vi "禹山电导率校准.vi"() -> ()   [LabVIEW 2016, in "斯坦道多参数.lvlib"]
uses:
  <vilib>/Utility/miscctls.llb/LVPointTypeDef.ctl
  <vilib>/Analysis/NI_AALBase.lvlib
  <vilib>/Analysis/NI_AALPro.lvlib
  <vilib>/Utility/config.llb/NI_LVConfig.lvlib
panel:
  out "第二点校准值":dbl
  out "第一点校准值":dbl
  out "最小值":sgl format="%.2g"
  out "最大值":sgl format="%.2g"
  in  "校准停止":bool
  in  "校准模式":enum16{"两点校准", "单点校准"}(ring)
  in  "标液2":dbl
  in  "标液1":dbl
  out "波形图表":sgl(graph) caption="历史曲线"
  out "温度测量值":dbl caption="温度"
  out "变异系数":dbl format="%.6g"
  out "standard deviation":dbl caption="标准差" format="%0.2f"
  out "mean":dbl caption="均值" format="%0.2f"
  out "提示":string
  in  "校准启动":bool
  out "测试值":dbl
  out "电极斜率":dbl
  out "电极零点":dbl
  # "电导率电极设定"
  # "℃"
  # "uS/cm"
  # "请选择校准模式:"
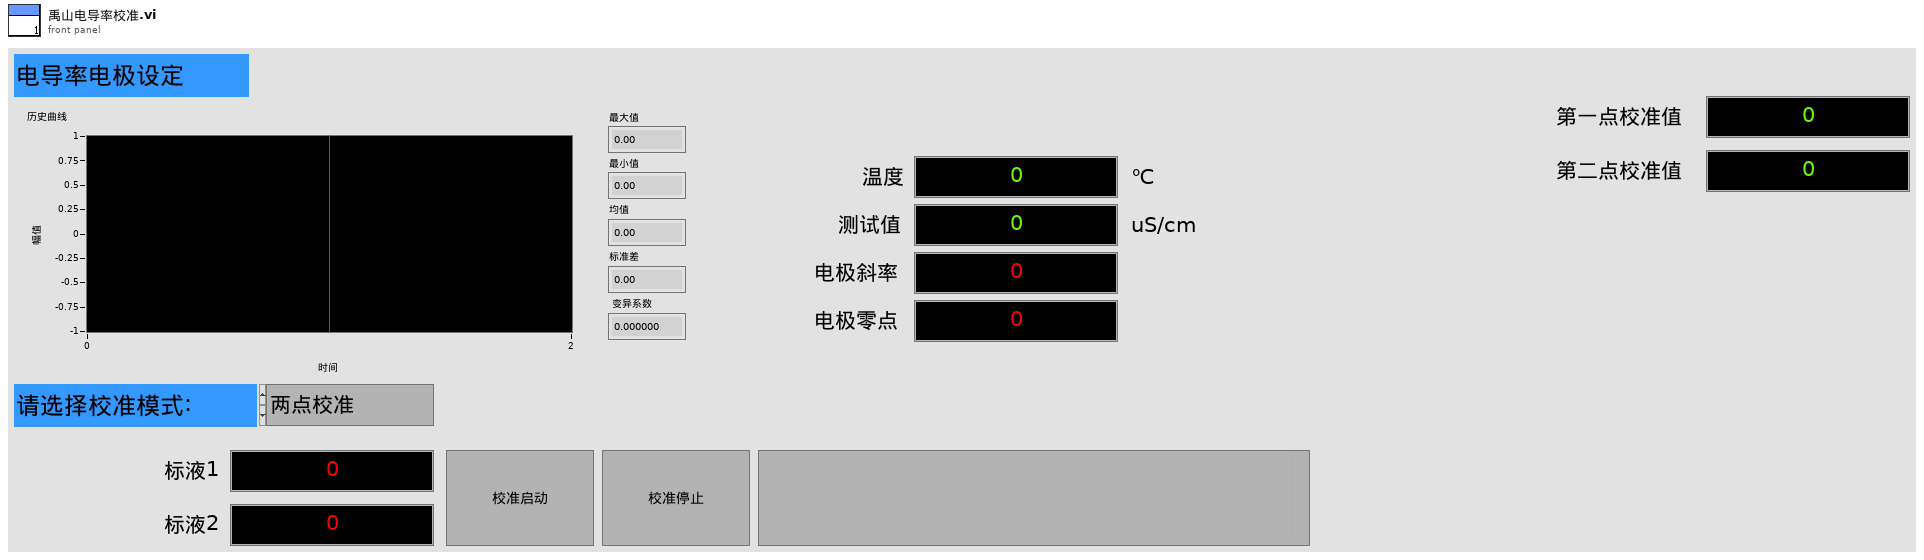
[diagram p1: front panel]
types:
  T1 = typedef "斯坦道多参数.lvlib/校准步骤.ctl" = enum16{"待机", "放置第一点标液", "第一点校准启动", "第一点校准写入", "第一点校准失败", "放置第二点标液", "第二点校准启动", "第二点校准写入", "第二点校准失败", "放置第三点标液", "第三点校准启动", "第三点校准写入", "第三点校准失败", "校准结果写入", "校准结束"}
  T2 = typedef "LVPointTypeDef.ctl" = cluster{"Horizontal":i16, "Vertical":i16}
  T3 = typedef "NI_LVConfig.lvlib/Config Data RefNum.ctl" = refnum<k1>
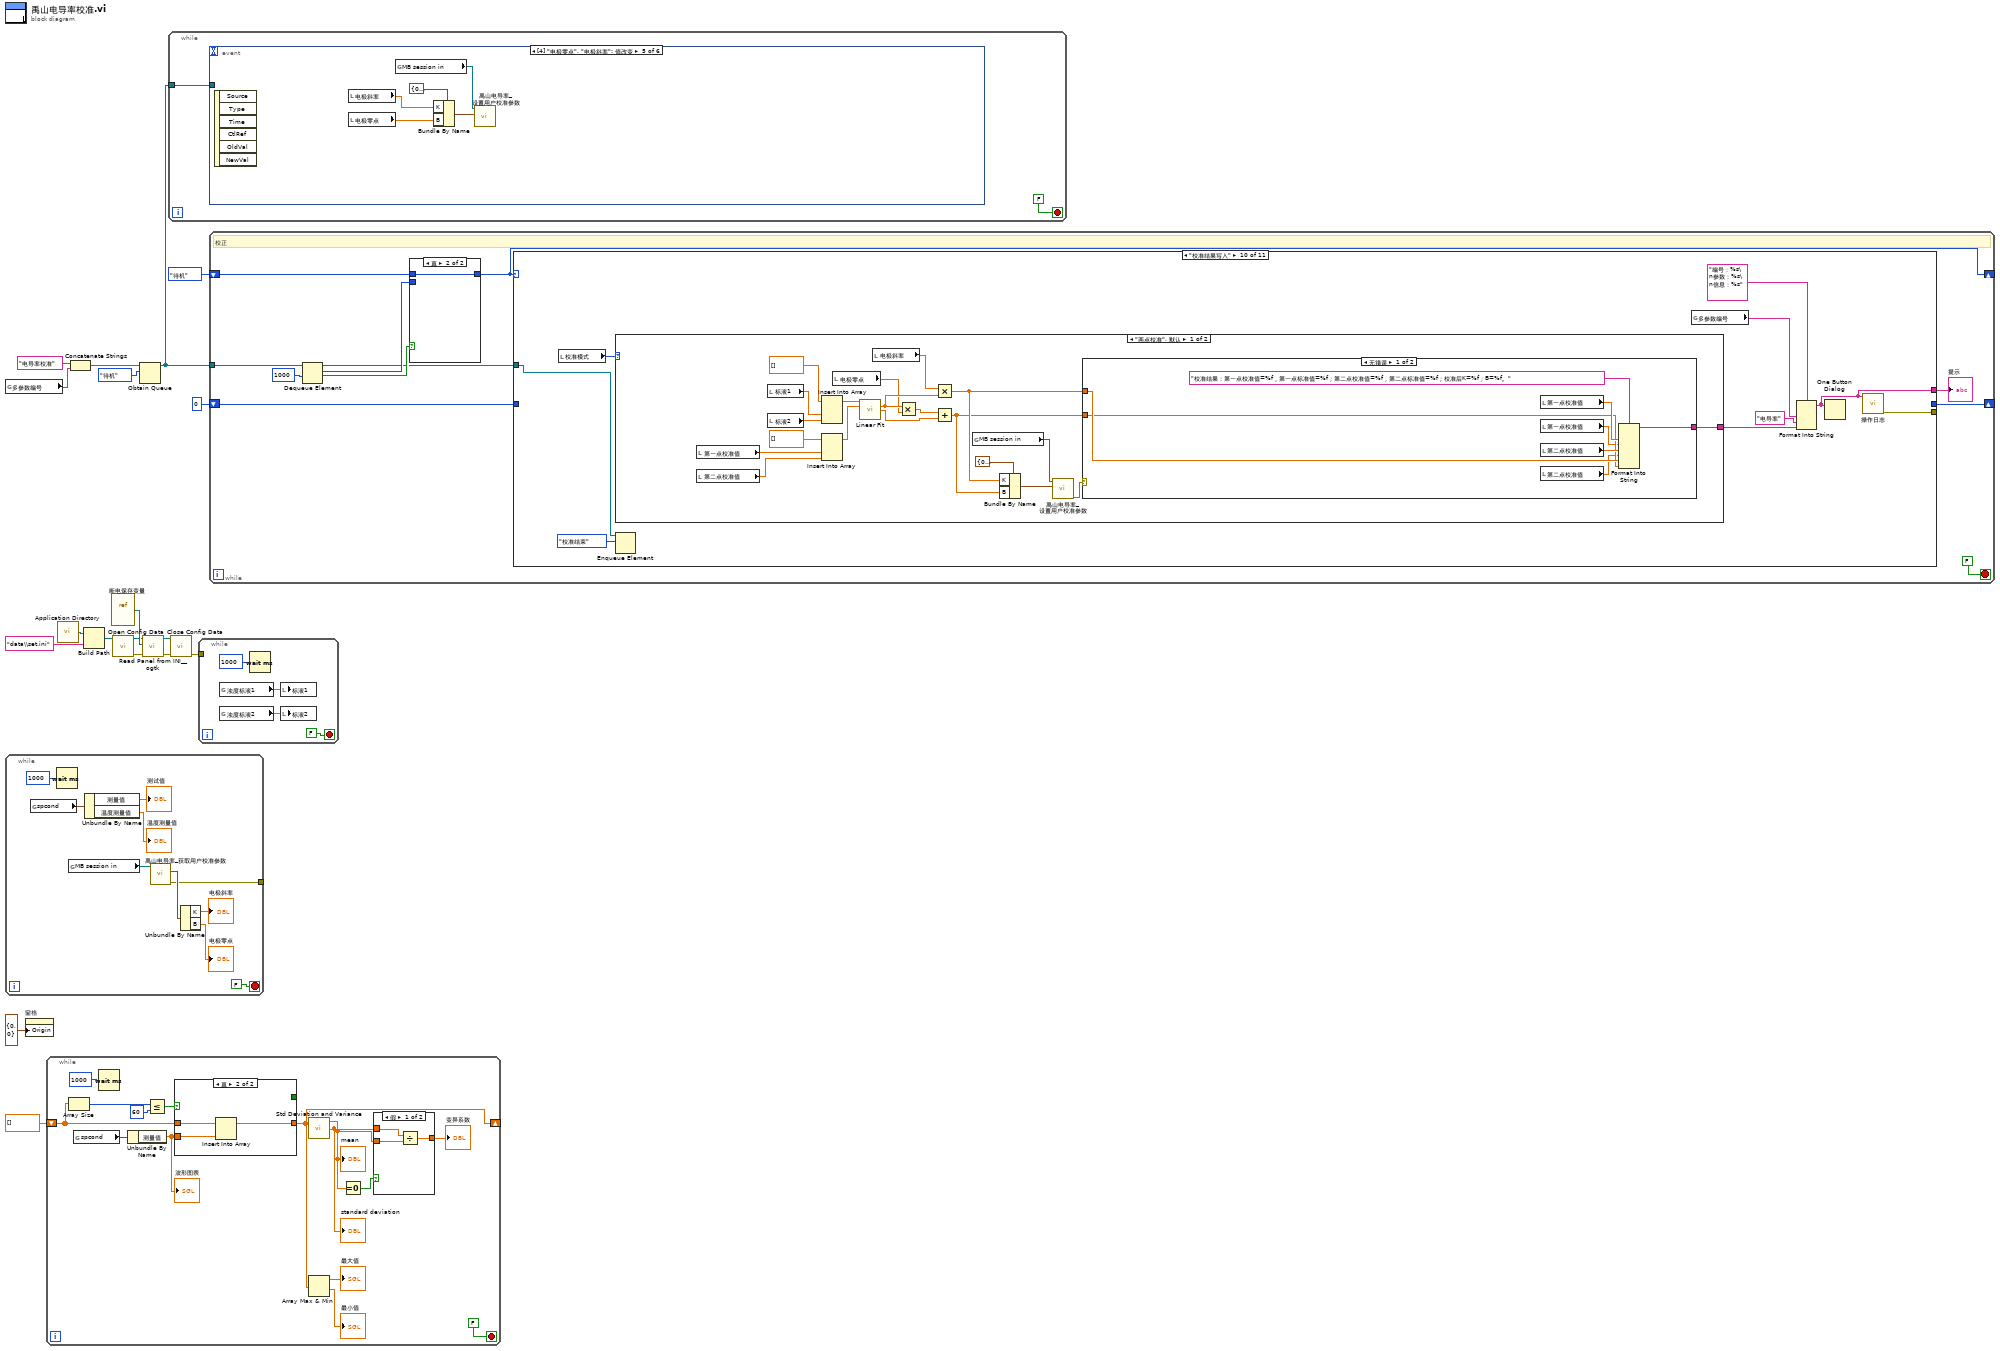
[diagram p0: block diagram]
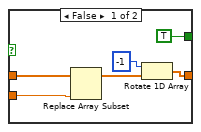
[diagram p3: hidden frame]
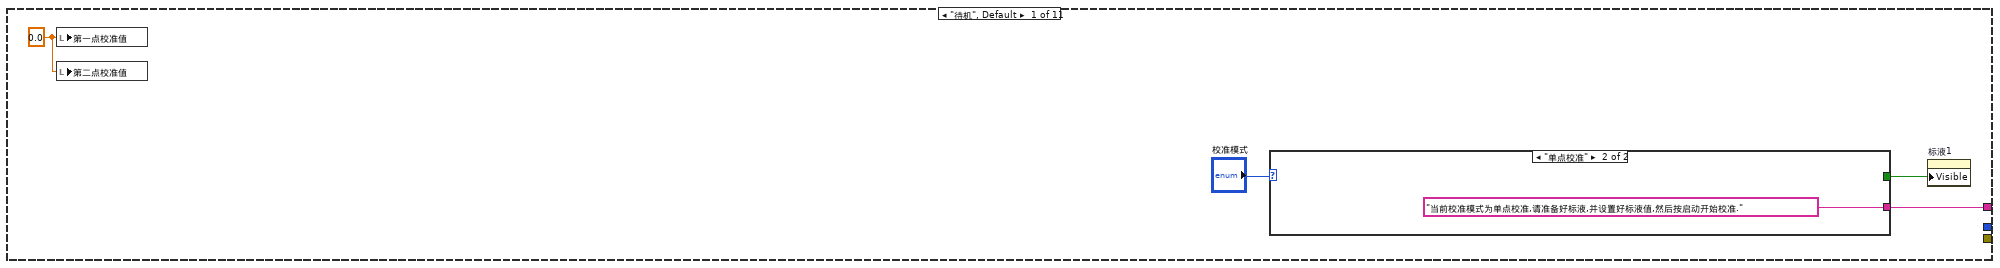
[diagram p5: hidden frame]
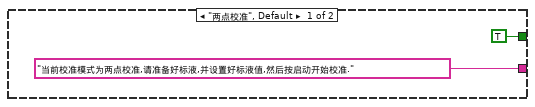
[diagram p6: hidden frame]
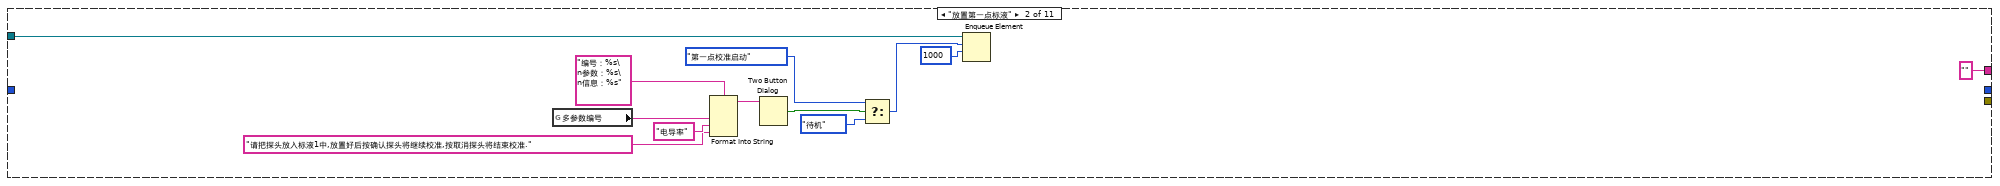
[diagram p7: hidden frame]
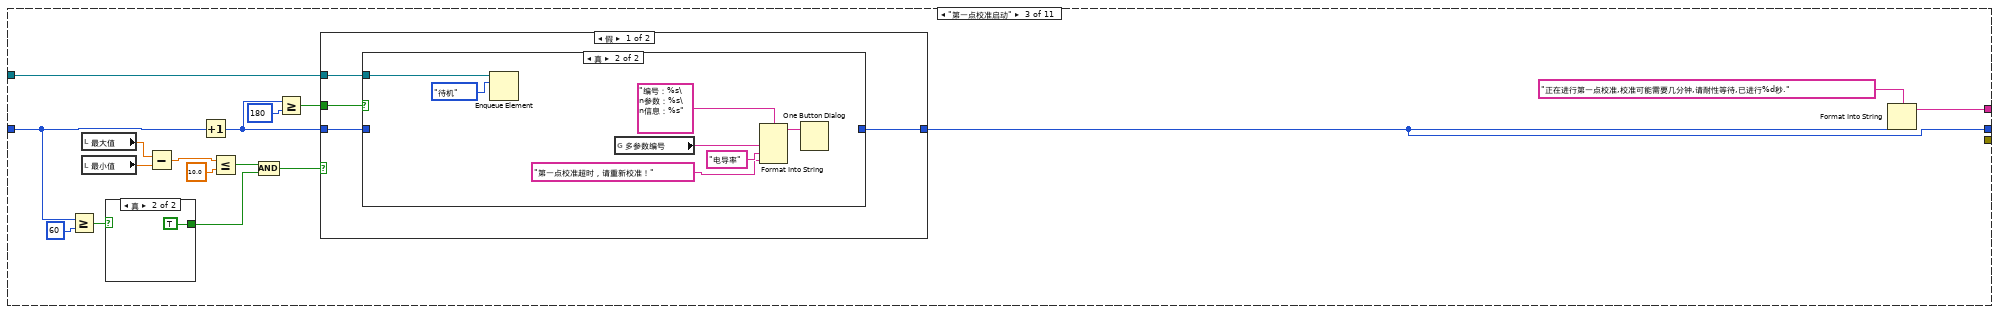
[diagram p8: hidden frame]
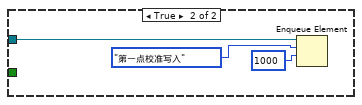
[diagram p10: hidden frame]
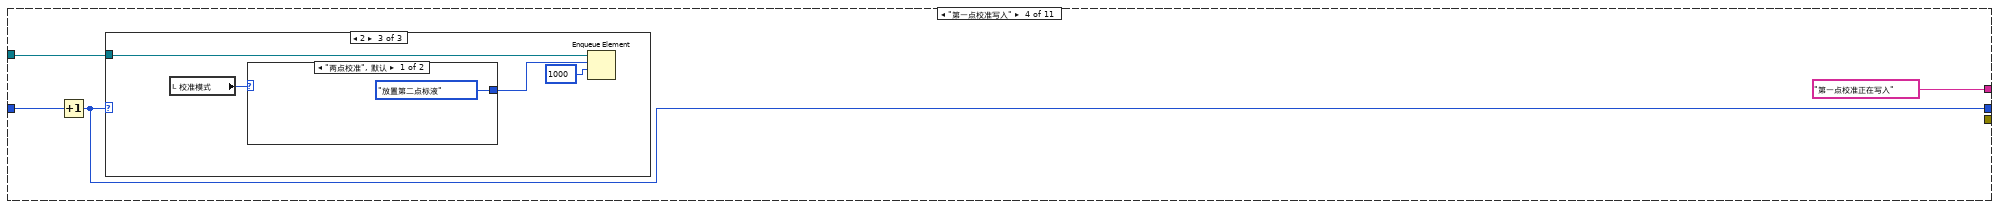
[diagram p12: hidden frame]
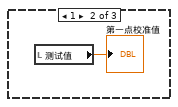
[diagram p14: hidden frame]
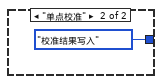
[diagram p15: hidden frame]
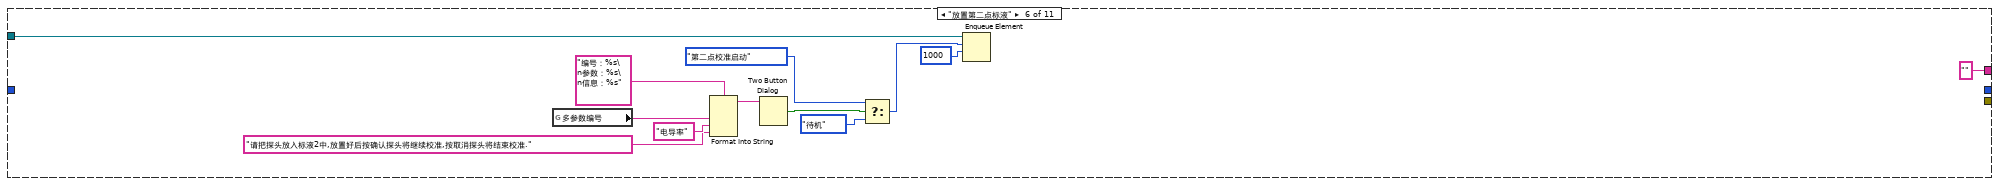
[diagram p17: hidden frame]
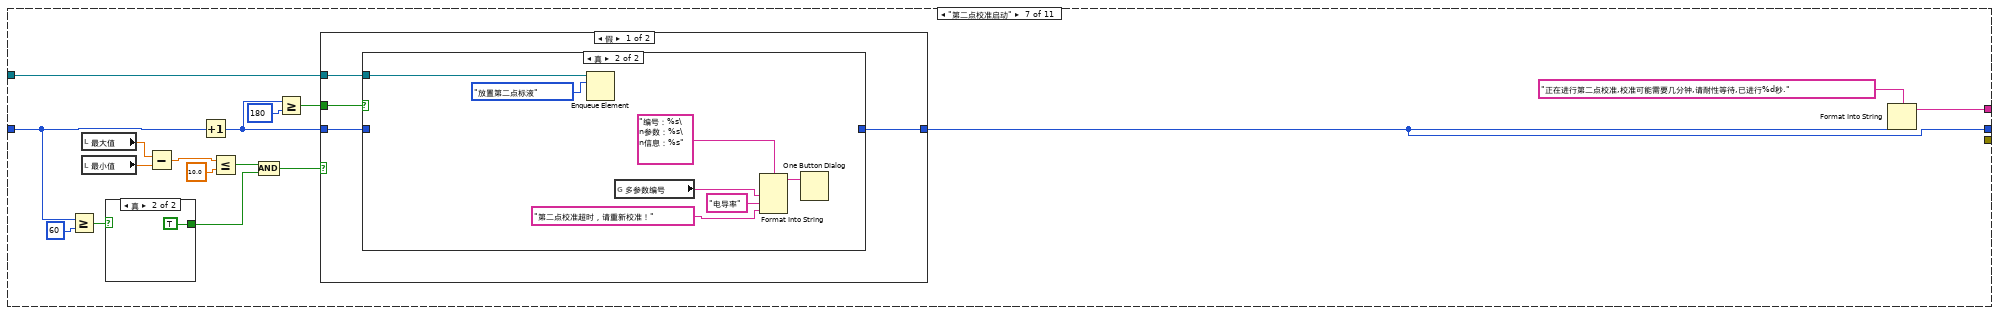
[diagram p18: hidden frame]
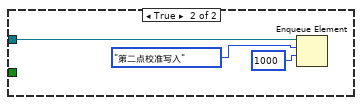
[diagram p20: hidden frame]
diagram:
  n1 = global read "多参数全局变量.vi" "多参数编号"() -> (w1:string)
  n2 = while {
    tunnel: [w23] -> _
    stop <- FALSE stop-if-true
    n3 = global read "禹山过程全局变量.vi" "spcond"() -> (w20:cluster{"温度测量值":sgl, "测量值":sgl, "错误标志":u16})
    n4 = Wait (ms)(milliseconds to wait=u32 1000 ("等待时间（毫秒）")) -> ()  [unwired: 1 out]
    n5 = global read "多参数全局变量.vi" "MB session in"() -> (w19:refnum<class "MB_Master.lvclass">)
    n6 = Unbundle By Name(w20) -> ("测量值"=→"测试值":sgl, "温度测量值"=→"温度测量值":sgl)
    n7 = call "禹山电导率_获取用户校准参数.vi"("MB session in"=w19) -> ("error out"=w23:errorcluster, "输出值"=w26:cluster{"K":sgl, "B":sgl})  [unwired: 8 in, 1 out]
    n8 = Unbundle By Name(w26) -> ("K"=→"电极斜率":sgl, "B"=→"电极零点":sgl)
  }
  n9 = property on="窗格" class="Pane"("Origin"=T2 {"Horizontal"=0, "Vertical"=0} ("原点")) -> ()  [unwired: 2 in, 2 out]
  n10 = while {
    shift-right: [w31] -> _
    shift-left: sgl[] [] -> [w39]
    stop <- FALSE stop-if-true
    n11 = Array Size(array=w39) -> (size(s)=w41:i32)
    n12 = global read "禹山过程全局变量.vi" "spcond"() -> (w33:cluster{"温度测量值":sgl, "测量值":sgl, "错误标志":u16})
    n13 = Wait (ms)(milliseconds to wait=u32 1000 ("等待时间（毫秒）")) -> ()  [unwired: 1 out]
    n14 = Unbundle By Name(w33) -> ("测量值"=w32:sgl)
    "波形图表" <- w32
    n15 = Less Or Equal?(x=w41, y=60) -> (x <= y?=w40:bool)
    n16 = case shown="真" w40 {
      tunnel: w39 -> [w52 w55]
      tunnel: w32 -> [w50 w54]
      tunnel: [w48 w53] -> w31
      tunnel: [TRUE _] -> _
      frame False {
        n17 = Replace Array Subset(array=w52, new element=w50) -> (w51:sgl[])  [unwired: 1 in]
        n18 = Rotate 1D Array(1:w51, 2:-1 ("n")) -> (0:w48:sgl[])
      }
      frame True {
        n19 = Insert Into Array(array=w55, new element=w54) -> (w53:sgl[])  [unwired: 1 in]
      }
    }
    n20 = call <vilib>:"Std Deviation and Variance.vi"("X"=w31) -> ("mean"=w34:dbl, "standard deviation"=w35:dbl)  [unwired: 1 in, 1 out]
    "standard deviation" <- w35
    "mean" <- w34
    n21 = Array Max & Min(array=w31) -> (max value=→"最大值":sgl, min value=→"最小值":sgl)  [unwired: 2 out]
    n22 = Equal To 0?(x=w34) -> (x = 0?=w38:bool)
    n23 = case shown="假" w38 {
      tunnel: w35 -> [w46 _]
      tunnel: [w45 _] -> w37
      tunnel: w34 -> [w44 _]
      frame False {
        n24 = Divide(x=w46, y=w44) -> (x/y=w45:dbl)
      }
      frame True {
      }
    }
    "变异系数" <- w37
  }
  n25 = call <vilib>:"Application Directory.vi"() -> ("Application Directory"=w8:path)
  n26 = Concatenate Strings("电导率校准" ("名称（未命名）"), w1) -> (w2:string)
  n27 = Build Path(base path=w8, name or relative path="data\\set.ini" ("名称或相对路径")) -> (appended path=w9:path)
  n28 = vi-ref "断电保存变量.vi"() -> (w11:refnum<vi>)
  n29 = call <vilib>:"Open Config Data.vi"("configuration file path"=w9) -> ("error out"=w5:errorcluster, "refnum"=w4:T3)  [unwired: 8 in, 1 out]
  n30 = Obtain Queue(name (unnamed)=w2, element data type=校准步骤."待机" ("枚举")) -> (queue out=w12:refnum<queue>)  [unwired: 3 in, 2 out]
  n31 = call <userlib>:"Read Panel from INI__ogtk.vi"("error in (no error)"=w5, "VI ref"=w11, "refnum"=w4) -> ("error out"=w7:errorcluster, "refnum out"=w6:T3)  [unwired: 7 in]
  n32 = while {
    tunnel: w12 -> [w56]
    stop <- FALSE stop-if-true
    n33 = event shown="[4] \"电极零点\", \"电极斜率\": 值改变" {
      selector: _ -> [_ _ _ _ _ _]
      dyn-events: _ -> [_ _ _ _ _ _]
      timeout: _ -> [_ _ _ _ _ _]
      tunnel: w56 -> [_ w59 w63 _ _ _]
      event Timeout {
        n34 = event-data() -> ()  [unwired: 1 in, 3 out]
      }
      event "校准启动": Value Change {
        n35 = event-data() -> ()  [unwired: 1 in, 6 out]
        n36 = Enqueue Element(queue=w59, element=校准步骤."放置第一点标液" ("元素")) -> ()  [unwired: 2 in, 3 out]
      }
      event "校准停止": Value Change {
        n37 = event-data() -> ()  [unwired: 1 in, 6 out]
        n38 = Flush Queue(queue=w63) -> (queue out=w60:refnum<queue>)  [unwired: 1 in, 2 out]
        n39 = Enqueue Element(queue=w60, element=校准步骤."待机" ("元素"), timeout in ms (-1)=1000 ("超时毫秒(-1)")) -> ()  [unwired: 1 in, 3 out]
      }
      event "电极零点", "电极斜率", "标液1", "标液2": Mouse Down {
        n40 = event-data() -> ("CtlRef"=w64:refnum<vi>)  [unwired: 1 in, 7 out]
        n41 = property class="DigNum (严格)"(reference=w64) -> (reference out=w65:refnum<vi>, "Value"=w66:dbl)  [unwired: 1 in, 1 out]
        n42 = call "数字键盘.vi"("OldNumber"=w66) -> ("NewNumber"=w67:dbl)  [unwired: 1 in]
        n43 = property class="DigNum (严格)"(reference=w65, "Val(Sgnl)"=w67) -> ()  [unwired: 1 in, 2 out]
      }
      event "电极零点", "电极斜率": Value Change {
        n44 = event-data() -> ()  [unwired: 1 in, 6 out]
        n45 = local read "电极斜率"() -> (w70:dbl)
        n46 = local read "电极零点"() -> (w69:dbl)
        n47 = global read "多参数全局变量.vi" "MB session in"() -> (w68:refnum<class "MB_Master.lvclass">)
        n48 = Bundle By Name(cluster=cluster{"K":sgl, "B":sgl} {"K"=0.0, "B"=0.0} ("用户校准参数"), "K"=w70, "B"=w69) -> (w71:cluster{"K":sgl, "B":sgl})
        n49 = call "禹山电导率_设置用户校准参数.vi"("用户校准参数"=w71, "MB session in"=w68) -> ()  [unwired: 8 in, 2 out]
      }
      event "标液1", "标液2": Value Change {
        n50 = event-data() -> ()  [unwired: 1 in, 6 out]
        n51 = flat-sequence {
          frame #0 {
            n52 = global write "断电保存变量.vi" "浊度标液1"("标液1") -> ()
            n53 = global write "断电保存变量.vi" "浊度标液2"("标液2") -> ()
          }
          frame #1 {
            n54 = call <vilib>:"Application Directory.vi"() -> ("Application Directory"=w84:path)
            n55 = Build Path(base path=w84, name or relative path="data\\set.ini" ("名称或相对路径")) -> (appended path=w83:path)
            n56 = call <vilib>:"Open Config Data.vi"("configuration file path"=w83) -> ("error out"=w87:errorcluster, "refnum"=w88:T3)  [unwired: 8 in, 1 out]
            n57 = vi-ref "断电保存变量.vi"() -> (w81:refnum<vi>)
            n58 = call <userlib>:"Write Panel to INI__ogtk.vi"("error in (no error)"=w87, "VI ref"=w81, "refnum"=w88) -> ("error out"=w85:errorcluster, "refnum out"=w86:T3)  [unwired: 7 in]
            n59 = call <vilib>:"Close Config Data.vi"("error in (no error)"=w85, "refnum"=w86) -> ("error out"=w77:errorcluster, "file path"=w78:path)  [unwired: 8 in]
            n60 = Open/Create/Replace File(file path (use dialog)=w78, error in=w77) -> (refnum out=w79:refnum<file>, error out=w80:errorcluster)  [unwired: 4 in, 1 out]
            n61 = Flush File(refnum=w79, error in=w80) -> (refnum out=w75:refnum<file>, error out=w76:errorcluster)
            n62 = Close File(refnum=w75, error in=w76) -> ()  [unwired: 2 out]
          }
        }
      }
    }
  }
  n63 = call <vilib>:"Close Config Data.vi"("error in (no error)"=w7, "refnum"=w6) -> ("error out"=w3:errorcluster)  [unwired: 8 in, 1 out]
  n64 = while {
    tunnel: w3 -> [_]
    stop <- FALSE stop-if-true
    n65 = global read "断电保存变量.vi" "浊度标液1"() -> (w90:dbl)
    n66 = global read "断电保存变量.vi" "浊度标液2"() -> (w89:dbl)
    n67 = Wait (ms)(milliseconds to wait=u32 1000 ("等待时间（毫秒）")) -> ()  [unwired: 1 out]
    n68 = local write "标液1"(w90) -> ()
    n69 = local write "标液2"(w89) -> ()
  }
  n70 = while "While循环" {
    shift-right: [w94] -> _
    shift-left: 校准步骤."待机" ("枚举") -> [w95]
    shift-right: [w101] -> _
    shift-left: 0 -> [w102]
    tunnel: w12 -> [w99]
    stop <- FALSE stop-if-true
    # "校正"
    n71 = Dequeue Element(queue=w99, timeout in ms (-1)=1000 ("超时毫秒(-1)")) -> (queue out=w93:refnum<queue>, element=w96:T1, timed out?=w97:bool)  [unwired: 1 in, 1 out]
    n72 = case shown="真" w97 {
      tunnel: w96 -> [w104 _]
      tunnel: [w104 w105] -> w94
      tunnel: w95 -> [_ w105]
      frame False {
      }
      frame True {
      }
    }
    n73 = case shown="\"校准结果写入\"" w94 {
      tunnel: [w109 "" ("提示") w140 "第一点校准正在写入" ("提示") _ "" ("提示") w196 "第二点校准正在写入" ("提示") _ w222 w276] -> w100
      tunnel: w102 -> [_ _ w134 w160 _ _ w190 w216 _ _ _]
      tunnel: [_ _ w125 w159 _ _ w181 w215 _ _ _] -> w101
      tunnel: w93 -> [_ w124 w128 w158 _ w180 w184 w214 _ w230 _]
      tunnel: [_ _ _ _ _ _ _ _ _ w227 _] -> _
      frame "待机", Default {
        w106 = 0.0 ("第一点校准值")
        n74 = local write "第一点校准值"(w106) -> ()
        n75 = local write "第二点校准值"(w106) -> ()
        n76 = case shown="\"单点校准\"" "校准模式" {
          tunnel: ["当前校准模式为两点校准,请准备好标液,并设置好标液值,然后按启动开始校准." ("提示") "当前校准模式为单点校准,请准备好标液,并设置好标液值,然后按启动开始校准." ("提示")] -> w109
          tunnel: [TRUE ("可见") _] -> w107
          frame "两点校准", Default {
          }
          frame "单点校准" {
          }
        }
        n77 = property on="标液1" class="DigNum (严格)"("Visible"=w107) -> ()  [unwired: 2 in, 2 out]
      }
      frame "放置第一点标液" {
        n78 = global read "多参数全局变量.vi" "多参数编号"() -> (w116:string)
        n79 = Format Into String(format string="编号：%s\n参数：%s\n信息：%s" ("格式字符串"), w116, "电导率" ("输入 2"), "请把探头放入标液1中,放置好后按确认探头将继续校准,按取消探头将结束校准." ("消息")) -> (resulting string=w113:string)  [unwired: 2 in, 1 out]
        n80 = Two Button Dialog(message=w113) -> (T button?=w122:bool)  [unwired: 2 in]
        n81 = Select(t=校准步骤."第一点校准启动" ("元素"), s=w122, f=校准步骤."待机" ("元素")) -> (s? t:f=w119:T1)
        n82 = Enqueue Element(queue=w124, element=w119, timeout in ms (-1)=1000 ("超时毫秒(-1)")) -> ()  [unwired: 1 in, 3 out]
      }
      frame "第一点校准启动" {
        n83 = Greater Or Equal?(x=w134, y=60) -> (x >= y?=w135:bool)
        n84 = local read "最大值"() -> (w131:sgl)
        n85 = local read "最小值"() -> (w132:sgl)
        n86 = case shown="真" w135 {
          tunnel: [_ TRUE] -> w133
          frame False {
          }
          frame True {
          }
        }
        n87 = Subtract(x=w131, y=w132) -> (x-y=w130:sgl)
        n88 = Increment(x=w134) -> (x+1=w126:i32)
        n89 = Less Or Equal?(x=w130, y=10.0) -> (x <= y?=w138:bool)
        n90 = And(x=w138, y=w133) -> (x .and. y?=w129:bool)
        n91 = Greater Or Equal?(x=w126, y=180) -> (x >= y?=w127:bool)
        n92 = case shown="假" w129 {
          tunnel: w128 -> [w144 w156]
          tunnel: w127 -> [w145 _]
          tunnel: w126 -> [w143 _]
          tunnel: [w142 _] -> w125
          frame False {
            n93 = case shown="真" w145 {
              tunnel: w144 -> [_ w153]
              tunnel: w143 -> [w146 _]
              tunnel: [w146 _] -> w142
              frame False {
              }
              frame True {
                n94 = Enqueue Element(queue=w153, element=校准步骤."待机" ("元素")) -> ()  [unwired: 2 in, 3 out]
                n95 = global read "多参数全局变量.vi" "多参数编号"() -> (w150:string)
                n96 = Format Into String(format string="编号：%s\n参数：%s\n信息：%s" ("格式字符串"), w150, "电导率" ("输入 2"), "第一点校准超时，请重新校准！" ("error source (\" \")")) -> (resulting string=w148:string)  [unwired: 2 in, 1 out]
                n97 = One Button Dialog(message=w148) -> ()  [unwired: 1 in, 1 out]
              }
            }
          }
          frame True {
            n98 = Enqueue Element(queue=w156, element=校准步骤."第一点校准写入" ("元素"), timeout in ms (-1)=1000 ("超时毫秒(-1)")) -> ()  [unwired: 1 in, 3 out]
          }
        }
        n99 = Format Into String(format string="正在进行第一点校准,校准可能需要几分钟,请耐性等待,已进行%d秒." ("格式字符串"), w125) -> (resulting string=w140:string)  [unwired: 2 in, 1 out]
      }
      frame "第一点校准写入" {
        n100 = Increment(x=w160) -> (x+1=w159:i32)
        n101 = case shown="2" w159 {
          tunnel: w158 -> [_ _ w166]
          frame 0, Default {
          }
          frame 1 {
            n102 = local read "测试值"() -> (→"第一点校准值":dbl)
          }
          frame 2 {
            n103 = local read "校准模式"() -> (w165:enum16{"两点校准", "单点校准"})
            n104 = case shown="\"两点校准\", 默认" w165 {
              tunnel: [校准步骤."放置第二点标液" ("元素") 校准步骤."校准结果写入" ("元素")] -> w164
              frame "两点校准", Default {
              }
              frame "单点校准" {
              }
            }
            n105 = Enqueue Element(queue=w166, element=w164, timeout in ms (-1)=1000 ("超时毫秒(-1)")) -> ()  [unwired: 1 in, 3 out]
          }
        }
      }
      frame "第一点校准失败" {
      }
      frame "放置第二点标液" {
        n106 = global read "多参数全局变量.vi" "多参数编号"() -> (w172:string)
        n107 = Format Into String(format string="编号：%s\n参数：%s\n信息：%s" ("格式字符串"), w172, "电导率" ("输入 2"), "请把探头放入标液2中,放置好后按确认探头将继续校准,按取消探头将结束校准." ("消息")) -> (resulting string=w169:string)  [unwired: 2 in, 1 out]
        n108 = Two Button Dialog(message=w169) -> (T button?=w178:bool)  [unwired: 2 in]
        n109 = Select(t=校准步骤."第二点校准启动" ("元素"), s=w178, f=校准步骤."待机" ("元素")) -> (s? t:f=w175:T1)
        n110 = Enqueue Element(queue=w180, element=w175, timeout in ms (-1)=1000 ("超时毫秒(-1)")) -> ()  [unwired: 1 in, 3 out]
      }
      frame "第二点校准启动" {
        n111 = Greater Or Equal?(x=w190, y=60) -> (x >= y?=w191:bool)
        n112 = local read "最大值"() -> (w187:sgl)
        n113 = local read "最小值"() -> (w188:sgl)
        n114 = case shown="真" w191 {
          tunnel: [_ TRUE] -> w189
          frame False {
          }
          frame True {
          }
        }
        n115 = Subtract(x=w187, y=w188) -> (x-y=w186:sgl)
        n116 = Increment(x=w190) -> (x+1=w182:i32)
        n117 = Less Or Equal?(x=w186, y=10.0) -> (x <= y?=w194:bool)
        n118 = And(x=w194, y=w189) -> (x .and. y?=w185:bool)
        n119 = Greater Or Equal?(x=w182, y=180) -> (x >= y?=w183:bool)
        n120 = case shown="假" w185 {
          tunnel: w184 -> [w200 w212]
          tunnel: w183 -> [w201 _]
          tunnel: w182 -> [w199 _]
          tunnel: [w198 _] -> w181
          frame False {
            n121 = case shown="真" w201 {
              tunnel: w200 -> [_ w209]
              tunnel: w199 -> [w202 _]
              tunnel: [w202 _] -> w198
              frame False {
              }
              frame True {
                n122 = Enqueue Element(queue=w209, element=校准步骤."放置第二点标液" ("元素")) -> ()  [unwired: 2 in, 3 out]
                n123 = global read "多参数全局变量.vi" "多参数编号"() -> (w206:string)
                n124 = Format Into String(format string="编号：%s\n参数：%s\n信息：%s" ("格式字符串"), w206, "电导率" ("输入 2"), "第二点校准超时，请重新校准！" ("error source (\" \")")) -> (resulting string=w204:string)  [unwired: 2 in, 1 out]
                n125 = One Button Dialog(message=w204) -> ()  [unwired: 1 in, 1 out]
              }
            }
          }
          frame True {
            n126 = Enqueue Element(queue=w212, element=校准步骤."第二点校准写入" ("元素"), timeout in ms (-1)=1000 ("超时毫秒(-1)")) -> ()  [unwired: 1 in, 3 out]
          }
        }
        n127 = Format Into String(format string="正在进行第二点校准,校准可能需要几分钟,请耐性等待,已进行%d秒." ("格式字符串"), w181) -> (resulting string=w196:string)  [unwired: 2 in, 1 out]
      }
      frame "第二点校准写入" {
        n128 = Increment(x=w216) -> (x+1=w215:i32)
        n129 = case shown="1" w215 {
          tunnel: w214 -> [_ _ w221]
          frame 0, Default {
          }
          frame 1 {
            n130 = local read "测试值"() -> (→"第二点校准值":dbl)
          }
          frame 2 {
            n131 = Enqueue Element(queue=w221, element=校准步骤."校准结果写入" ("元素"), timeout in ms (-1)=1000 ("超时毫秒(-1)")) -> ()  [unwired: 1 in, 3 out]
          }
        }
      }
      frame "第二点校准失败" {
      }
      frame "校准结果写入" {
        n132 = local read "校准模式"() -> (w228:enum16{"两点校准", "单点校准"})
        n133 = case shown="\"两点校准\", 默认" w228 {
          tunnel: [w238 w264] -> w223
          frame "两点校准", Default {
            n134 = local read "第一点校准值"() -> (w249:dbl)
            n135 = local read "第二点校准值"() -> (w248:dbl)
            n136 = local read "标液1"() -> (w246:dbl)
            n137 = local read "标液2"() -> (w245:dbl)
            n138 = Insert Into Array(array=dbl[] [] ("Weight"), new element #1=w246, new element #2=w245) -> (w244:dbl[])  [unwired: 1 in]
            n139 = Insert Into Array(array=dbl[] [] ("Weight"), new element #1=w249, new element #2=w248) -> (w243:dbl[])  [unwired: 1 in]
            n140 = local read "电极零点"() -> (w234:dbl)
            n141 = call <vilib>:"Linear Fit.vi"("Y"=w244, "X"=w243) -> ("slope"=w235:dbl, "intercept"=w232:dbl)  [unwired: 9 in, 3 out]
            n142 = local read "电极斜率"() -> (w237:dbl)
            n143 = Multiply(x=w235, y=w234) -> (x*y=w233:dbl)
            n144 = Multiply(x=w237, y=w235) -> (x*y=w236:dbl)
            n145 = Add(x=w233, y=w232) -> (x+y=w231:dbl)
            n146 = global read "多参数全局变量.vi" "MB session in"() -> (w242:refnum<class "MB_Master.lvclass">)
            n147 = Bundle By Name(cluster=cluster{"K":sgl, "B":sgl} {"K"=0.0, "B"=0.0} ("用户校准参数"), "K"=w236, "B"=w231) -> (w241:cluster{"K":sgl, "B":sgl})
            n148 = call "禹山电导率_设置用户校准参数.vi"("用户校准参数"=w241, "MB session in"=w242) -> ("error out"=w239:errorcluster)  [unwired: 8 in, 1 out]
            n149 = case shown="无错误" w239 {
              tunnel: w236 -> [w256 _]
              tunnel: w231 -> [w255 _]
              tunnel: [w254 "校准失败"] -> w238
              frame No Error {
                n150 = local read "第一点校准值"() -> (w257:dbl)
                n151 = local read "第一点校准值"() -> (w252:dbl)
                n152 = local read "第二点校准值"() -> (w258:dbl)
                n153 = local read "第二点校准值"() -> (w251:dbl)
                n154 = Format Into String(format string="校准结果：第一点校准值=%f，第一点标准值=%f；第二点校准值=%f，第二点标准值=%f；校准后K=%f；B=%f。" ("提示"), w257, w252, w258, w251, w256, w255) -> (resulting string=w254:string)  [unwired: 2 in, 1 out]
              }
              frame Error {
              }
            }
          }
          frame "单点校准" {
            n155 = local read "第一点校准值"() -> (w262:dbl)
            n156 = local read "标液2"() -> (w261:dbl)
            n157 = local read "电极斜率"() -> (w263:dbl)
            n158 = Subtract(x=w261, y=w262) -> (x-y=w260:dbl)
            n159 = global read "多参数全局变量.vi" "MB session in"() -> (w268:refnum<class "MB_Master.lvclass">)
            n160 = Bundle By Name(cluster=cluster{"K":sgl, "B":sgl} {"K"=0.0, "B"=0.0} ("用户校准参数"), "K"=w263, "B"=w260) -> (w267:cluster{"K":sgl, "B":sgl})
            n161 = call "禹山电导率_设置用户校准参数.vi"("用户校准参数"=w267, "MB session in"=w268) -> ("error out"=w265:errorcluster)  [unwired: 8 in, 1 out]
            n162 = case shown="无错误" w265 {
              tunnel: w263 -> [w273 _]
              tunnel: w260 -> [w272 _]
              tunnel: [w271 "校准失败"] -> w264
              frame No Error {
                n163 = local read "第一点校准值"() -> (w274:dbl)
                n164 = local read "标液2"() -> (w269:dbl)
                n165 = Format Into String(format string="校准结果：校准值=%f，标准值=%f，校准后K=%f，B=%f。" ("提示"), w274, w269, w273, w272) -> (resulting string=w271:string)  [unwired: 2 in, 1 out]
              }
              frame Error {
              }
            }
          }
        }
        n166 = Enqueue Element(queue=w230, element=校准步骤."校准结束" ("元素")) -> ()  [unwired: 2 in, 3 out]
        n167 = global read "多参数全局变量.vi" "多参数编号"() -> (w225:string)
        n168 = Format Into String(format string="编号：%s\n参数：%s\n信息：%s" ("格式字符串"), w225, "电导率" ("输入 2"), w223) -> (resulting string=w222:string)  [unwired: 2 in, 1 out]
        n169 = One Button Dialog(message=w222) -> ()  [unwired: 1 in, 1 out]
        n170 = call "操作日志.vi"("日志信息"=w222) -> ("error out"=w227:errorcluster)  [unwired: 10 in]
      }
      frame "校准结束" {
        n171 = local read "提示"() -> (w276:string)
      }
    }
    "提示" <- w100
  }
